vi "hse-config-ini_ReadKey.vi"(8 "error in (no error)":errorcluster, 9 "Key":string, 10 "Section":string, 11 "hse-config-ini in":refnum<class "hse-config-ini.lvclass">) -> (0 "error out":errorcluster, 2 "String":string, 3 "hse-config-ini out":refnum<class "hse-config-ini.lvclass">)   [LabVIEW 2014, in "hse-config-ini.lvclass"]
uses:
  hse-config-ini.lvclass
  hse-configuration.lvclass/hse-configuration.ctl
  hse-configuration_ReadDataDirectory.vi
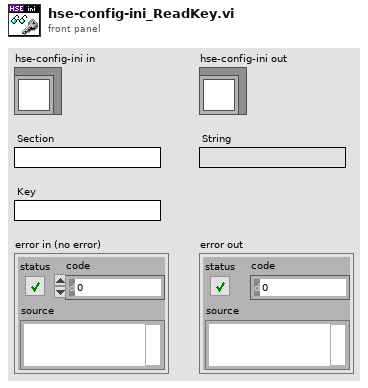
[diagram p1: front panel]
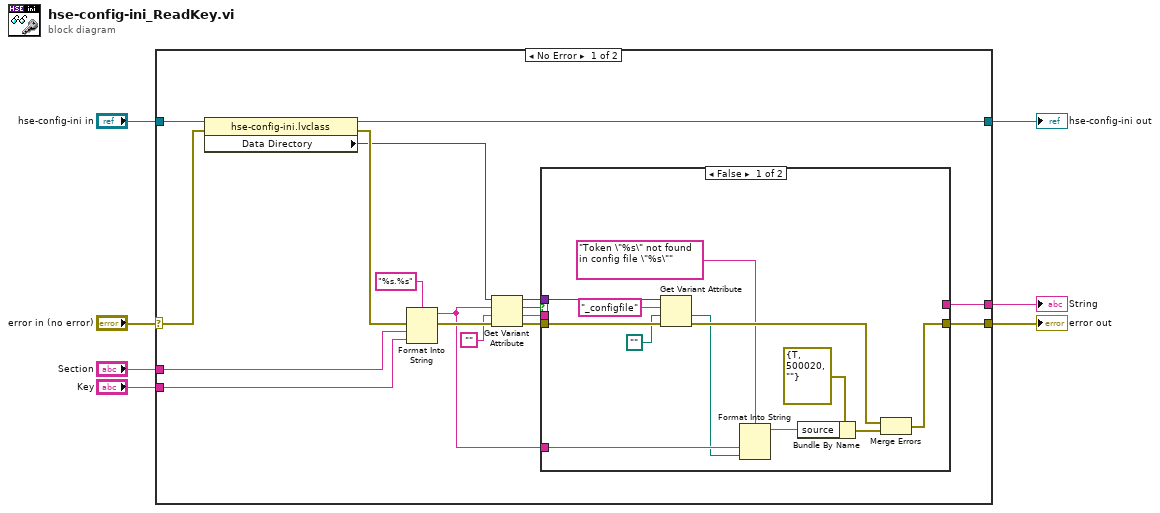
[diagram p0: block diagram]
diagram:
  n1 = case shown="No Error" "error in (no error)" {
    selector: "error in (no error)" -> [w18 w39]
    tunnel: [w24 w39] -> w7
    tunnel: [w11 _] -> w6
    tunnel: "Key" -> [w17 _]
    tunnel: "Section" -> [w16 _]
    tunnel: [w14 w40] -> w2
    tunnel: "hse-config-ini in" -> [w13 w40]
    frame No Error {
      n2 = property class="hse-config-ini.lvclass"(reference=w13, error in=w18) -> (reference out=w14:refnum<class "hse-config-ini.lvclass">, error out=w19:errorcluster, "Data Directory"=w15:variant)
      n3 = Format Into String(format string="%s.%s", error in=w19, w16, w17) -> (resulting string=w9:string, error out=w20:errorcluster)  [unwired: 1 in]
      n4 = Get Variant Attribute(Variant=w15, name=w9, default value (empty Variant)="", error in=w20) -> (duplicate Variant=w8:variant, found=w22:bool, value=w12:string, error out=w23:errorcluster)
      n5 = case shown="False" w22 {
        tunnel: [w32 w38] -> w24
        tunnel: w9 -> [w34 _]
        tunnel: w23 -> [w30 w38]
        tunnel: [_ w37] -> w11
        tunnel: w12 -> [_ w37]
        tunnel: w8 -> [w31 _]
        frame False {
          n6 = Get Variant Attribute(Variant=w31, name="_configfile", default value (empty Variant)=path "", error in=w30) -> (value=w27:path, error out=w29:errorcluster)  [unwired: 2 out]
          n7 = Format Into String(format string="Token \"%s\" not found in config file \"%s\"", w34, w27) -> (resulting string=w35:string)  [unwired: 2 in, 1 out]
          n8 = Bundle By Name(cluster=errorcluster {"status"=TRUE, "code"=500020, "source"=""} ("t"), "source"=w35) -> (w33:errorcluster)
          n9 = Merge Errors(w29, w33) -> (w32:errorcluster)
        }
        frame True {
        }
      }
    }
    frame Error {
    }
  }
  "error out" <- w7
  "String" <- w6
  "hse-config-ini out" <- w2
